vi "stop_read.vi"(6 "timeout (0)":i32, 7 "references":T1, 8 "error in (no error)":errorcluster) -> (0 "error out":errorcluster, 3 "stop?":bool)   [LabVIEW 2015, in "lv-recipe-machine.lvlib"]
doc: "This VI will return the most recent value for the stop notifier. It can be used to create a global \"Stop\" for all running loops for a specific module."
uses:
  lv-recipe-machine.lvlib
  public/_controls/references.ctl
  public/_controls/input.ctl
  public/_controls/input_command.ctl
  public/_controls/output.ctl
  public/_controls/transition.ctl
  public/_controls/data.ctl
  public/_controls/configuration.ctl
  public/_controls/recipe_data.ctl
  public/_controls/mode.ctl
  public/_controls/manual_state.ctl
  public/_controls/automatic_state.ctl
  public/_controls/timer.ctl
  public/_controls/recipe_step.ctl
  public/_controls/change.ctl
  public/_controls/status.ctl
  public/_controls/error.ctl
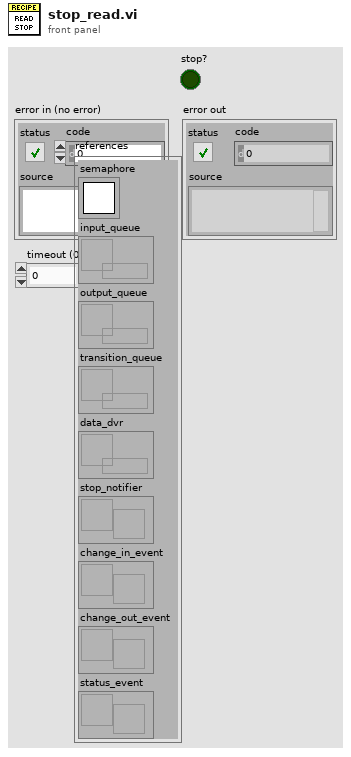
[diagram p1: front panel]
types:
  T1 = typedef "lv-recipe-machine.lvlib/references.ctl" = cluster{"semaphore":T2, "input_queue":refnum<queue>, "output_queue":refnum<queue>, "transition_queue":refnum<queue>, "data_dvr":refnum<data-value>, "stop_notifier":refnum<notifier>, "change_in_event":refnum<user-event>, "change_out_event":refnum<user-event>, "status_event":refnum<user-event>}
  T2 = typedef "Semaphore RefNum" = refnum<k1>
  T3 = typedef "lv-recipe-machine.lvlib/error.ctl" = enum16{"<error>", "bad_command", "command_queue_timeout", "stop_notifier_timeout", "die_command_timeout", "not_in_manual_mode", "not_in_automatic_mode", "not_in_automatic_idle", "not_in_automatic_running", "not_in_automatic_paused", "automatic_step_not_found", "manual_action_not_found", "automatic_not_transition_vi", "transition_step_not_found", "unsupported_vi_type", "<null>"}
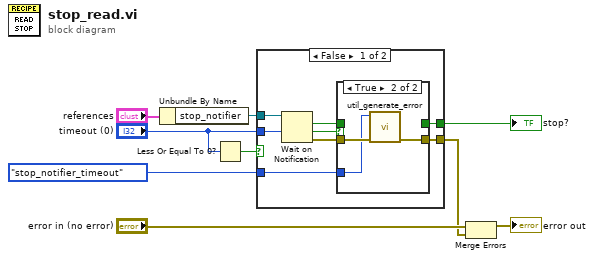
[diagram p0: block diagram]
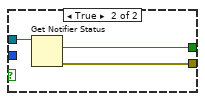
[diagram p3: hidden frame]
diagram:
  n1 = Unbundle By Name("references") -> ("stop_notifier"=w6:refnum<notifier>)
  n2 = Less Or Equal To 0?(x="timeout (0)") -> (x <= 0?=w7:bool)
  n3 = case shown="False" w7 {
    tunnel: "timeout (0)" -> [w17 _]
    tunnel: w6 -> [w16 w25]
    tunnel: [w11 w24] -> w8
    tunnel: [w12 w23] -> w3
    tunnel: error."stop_notifier_timeout" ("Error") -> [w10 _]
    frame False {
      n4 = Wait on Notification(notifier=w16, timeout in ms (-1)=w17) -> (notification=w15:bool, timed out?=w14:bool, error out=w13:errorcluster)  [unwired: 2 in, 1 out]
      n5 = case shown="True" w14 {
        tunnel: w15 -> [w19 _]
        tunnel: w13 -> [w18 w22]
        tunnel: [w18 w21] -> w12
        tunnel: [w19 _] -> w11
        tunnel: w10 -> [_ w20]
        frame False {
        }
        frame True {
          n6 = call "util_generate_error.vi"("error in (no error)"=w22, "error"=w20) -> ("error out"=w21:errorcluster)  [unwired: 9 in]
        }
      }
    }
    frame True {
      n7 = Get Notifier Status(notifier=w25) -> (current notification=w24:bool, error out=w23:errorcluster)  [unwired: 1 in, 3 out]
    }
  }
  "stop?" <- w8
  n8 = Merge Errors("error in (no error)", w3) -> (→"error out":errorcluster)
